vi "AG34980A_Configure_DC_Current.vi"(0 "VISA resource name":refnum<visa-resource-name>, 5 "Range (3:Auto)":T2(ring)=enum."Auto", 7 "Resolution (5:Default) 2":T1(ring)=enum."Default", 9 "Autozero (0:ON)":enum16{"On", "Off", "Once"}(ring), 11 "error in (no error)":errorcluster) -> (4 "VISA resource name out":refnum<visa-resource-name>, 15 "error out":errorcluster)   [LabVIEW 2022 SP3, in "DMM_Keysight_34980A.lvlib" / "DMM_Keysight_34980A.lvclass"]
doc: "This VI allows you to control various settings for performing DC current measurements. You can independently control the range, resolution, and autozero settings."
uses:
  DMM_Keysight_34980A.lvclass
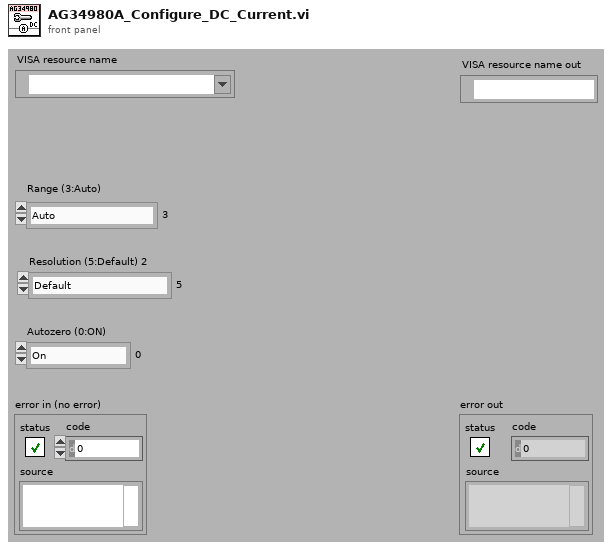
[diagram p1: front panel]
types:
  T1 = enum16{"4 1/2", "5 1/2", "6 1/2", "Least", "Highest", "Default"}
  T2 = enum16{"10 mA", "100 mA", "1 A", "Auto", "Minimum", "Maximum", "Default"}
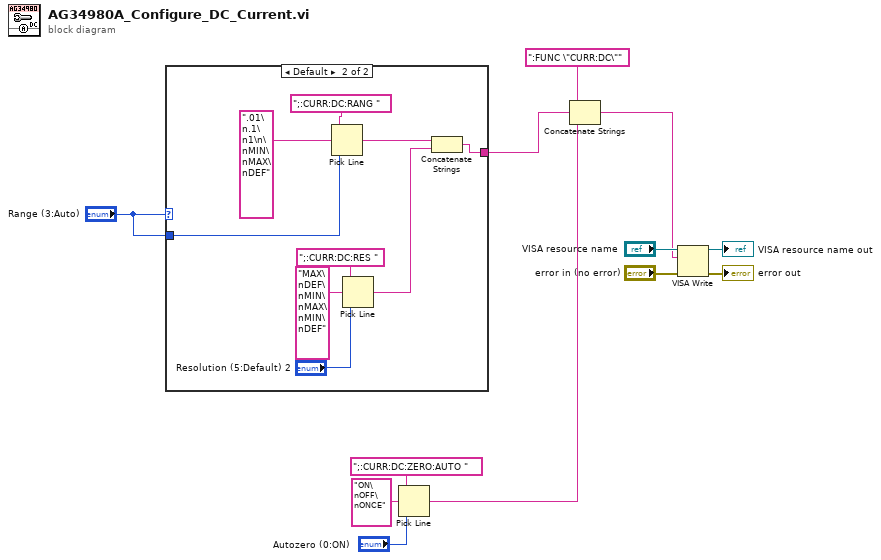
[diagram p0: block diagram]
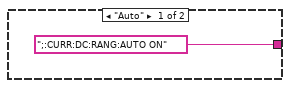
[diagram p2: hidden frame]
diagram:
  n1 = case shown="Default" "Range (3:Auto)" {
    tunnel: [";:CURR:DC:RANG:AUTO ON" ("output string") w14] -> w4
    tunnel: "Range (3:Auto)" -> [_ w20]
    frame "Auto" {
    }
    frame Default {
      n2 = Pick Line(string ("")=";:CURR:DC:RANG ", multi-line string=".01\n.1\n1\n\nMIN\nMAX\nDEF", line index=w20) -> (output string=w16:string)
      n3 = Pick Line(string ("")=";:CURR:DC:RES ", multi-line string="MAX\nDEF\nMIN\nMAX\nMIN\nDEF", line index="Resolution (5:Default) 2") -> (output string=w15:string)
      n4 = Concatenate Strings(w16, w15) -> (w14:string)
    }
  }
  n5 = Pick Line(string ("")=";:CURR:DC:ZERO:AUTO ", multi-line string="ON\nOFF\nONCE", line index="Autozero (0:ON)") -> (output string=w1:string)
  n6 = Concatenate Strings(":FUNC \"CURR:DC\"", w4, w1) -> (w2:string)
  n7 = VISA Write(VISA resource name="VISA resource name", write buffer=w2, error in (no error)="error in (no error)") -> (VISA resource name out=→"VISA resource name out":refnum<visa-resource-name>, error out=→"error out":errorcluster)  [unwired: 1 out]
